vi "Drivetrain Loop.vi"(6 "Reset the clock":bool, 8 "In 4":dbl, 9 "In 3":dbl, 10 "In 2":dbl, 11 "In 1":dbl) -> (0 "Out 4":dbl, 1 "Out 3":dbl, 2 "Out 2":dbl, 3 "Out 1":dbl)   [LabVIEW 2015]
uses:
  Common Code/Drivetrain Modes.ctl
  Robot Global Data.vi
  <vilib>/Rock Robotics/WPI/Solenoid/Deprecated/WPI_SolenoidSetBool.vi
panel:
  out "Modes":T1=enum."Ball Vision Targeting"
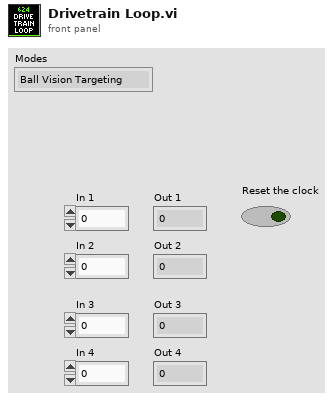
[diagram p1: front panel]
types:
  T1 = typedef "Drivetrain Modes.ctl" = enum16{"Climb", "Manual", "Ball Vision Targeting", "Goal Vision Targeting", "PID Distance Drive", "Hybrid"}
  T2 = typedef "Drivetrain Commands.ctl" = cluster{"Y Power":dbl, "Turn Power":dbl, "1st Gear?":bool, "Modes":T1, "Heading Target":dbl, "X Max Speed":dbl, "Y Max Speed":dbl, "X Min Speed":dbl, "Y Min Speed":dbl, "Y Target":dbl, "Max Accel":dbl, "Max Velocity":dbl}
  T3 = typedef "Dashboard Control Data.ctl" = cluster{"Shooter Presets":T4, "Encoder Control":T6, "Steer PID output":cluster{"output high":dbl, "output low":dbl}, " Steer PID gains":cluster{"proportional gain (Kc)":dbl, "integral time (Ti, min)":dbl, "derivative time (Td, min)":dbl}, "Drivetrain Settings":T7, "Vision Packet":T8, "Dashboard Drivetrain Command":T9, "Info/Command Cluster":T11, "Ball Vision Packet":T12, "Intake Presets":T14, "Intake Encoder Control":T16, "Climb Presets":T17, "Ultrasonic Limit":dbl, "Roll Limit":dbl, "Pitch Limit":dbl, "Goal Output Range":cluster{"output high":dbl, "output low":dbl}}
  T4 = typedef "Shooter Presets.ctl" = cluster{"Batter Shot":T5, "Deep Middle Shot":T5, "Manual Shot":T5, "Left Ticks Per Rotation":dbl, "Right Ticks Per Rotation":dbl, "Low Bar Shot":T5, "Shooter RPM Tolerance":dbl, "IIR Filter Power":dbl, "Trigger Power":dbl, "Fire from Load Delay":i32, "Angle Pot M":dbl, "Angle Pot B":dbl, "Shooter Length":dbl, "String Pot Dist":dbl, "Angle PID gains":cluster{"proportional gain (Kc)":dbl, "integral time (Ti, min)":dbl, "derivative time (Td, min)":dbl}, "Angle Motor Output":cluster{"output high":dbl, "output low":dbl}, "Shooter Angle Tolerance":dbl, "Vision Shoot x^2":dbl, "Vision Shoot x":dbl, "Dist from Axis Cam to Pivot":dbl, "High Goal Center Height":dbl, "Feed Forward Max Accel":dbl, "Feed Forward Kv":dbl, "Backwards Trigger":dbl, "Shot Finish Delay (ms)":dbl, "Angle Max Current":dbl, "Angle Current Trip Time":dbl, "Shooter Intake Angle":dbl, "Vision Shoot c":dbl, "Reset?":bool, "Servo Release Delay":dbl, "Servo Idle Angle":i32, "Servo Hold Angle":i32, "Angle Pot x^2":dbl, "Angle Pot x":dbl, "Angle Pot c":dbl, "Ignore Angle?":bool}
  T5 = typedef "Shot Presets.ctl" = cluster{"Left Wheel RPM":dbl, "Right Wheel RPM":dbl, "Angle":dbl}
  T6 = typedef "Encoder Control.ctl" = cluster{"Right Tick Constant":dbl, "Left Tick Constant":dbl, "Reset?":bool, "Y Dist":cluster{"PID gains":cluster{"proportional gain (Kc)":dbl, "integral time (Ti, min)":dbl, "derivative time (Td, min)":dbl}}, "Y Stop Thresh":dbl, "Y Stop Speed":dbl}
  T7 = typedef "Drivetrain Settings.ctl" = cluster{"Gyro Tolerance":dbl, "Throttle Ramp (ms)":dbl, "Angular rate compensation":bool, "Throttle to Rate Scale":dbl, "Rate compensation gain":dbl, "Kv":dbl, "Ka":dbl, "Feed Forward P":dbl, "Feed Forward D":dbl, "Goal Vision PID gains":cluster{"proportional gain (Kc)":dbl, "integral time (Ti, min)":dbl, "derivative time (Td, min)":dbl}, "Goal Detection Window":dbl}
  T8 = typedef "Goal Vision Packet.ctl" = cluster{"Distance":dbl, "Center X":dbl, "Center Y":dbl, "Found Target?":bool}
  T9 = typedef "Dashboard Drivetrain Command.ctl" = cluster{"Drivetrain Vision":T10}
  T10 = typedef "Drivetrain Vision.ctl" = cluster{"Goal Window":dbl, "Ball Window":dbl}
  T11 = typedef "Ball Tracking Command Cluster.ctl" = cluster{"Distance to Ball":dbl, "Desired Angle":dbl, "Command":enum16{"Turn to Ball", "Turn to Angle", "Get Distance"}, "Pixels from Center":dbl}
  T12 = typedef "Ball Vision Packet.ctl" = cluster{"Ball Detected?":bool, "Distance to Ball":dbl, "Desired Angle":dbl, "Pixels from Center":dbl, "Tracking mode":T13}
  T13 = typedef "Tracking Mode.ctl" = enum16{"Turn to Ball", "Turn to Angle"}
  T14 = typedef "Intake Presets.ctl" = cluster{"Intake Speed":dbl, "Outake Speed":dbl, "Low Height":dbl, "Half Height":dbl, "Full Height":dbl, "Angle Speed":dbl, "Fast Angle":dbl, "Encoder Scale":dbl, "Load Height":dbl, "Output Range":T15, "Rotation Power Max/Min":dbl, "MaxCurrent":dbl, "Intake Trip Time":dbl, "Idle Height":dbl, "Max Height":dbl, "Reset Encoders?":bool, "PID gains":cluster{"proportional gain (Kc)":dbl, "integral time (Ti, min)":dbl, "derivative time (Td, min)":dbl}}
  T15 = typedef "Drivetrain Output Range.ctl" = cluster{"output high":dbl, "output low":dbl}
  T16 = typedef "IntakeEcoderControl.ctl" = cluster{"Arm Tick Constant":dbl, "Reset?":bool, "Y Dist":cluster{"PID gains":cluster{"proportional gain (Kc)":dbl, "integral time (Ti, min)":dbl, "derivative time (Td, min)":dbl}}, "Y Stop Thresh":dbl, "Y Stop Speed":dbl}
  T17 = typedef "Climb Presets.ctl" = cluster{"Pull Power":dbl, "Unpin Power":dbl, "Time to Hold":dbl}
  T18 = typedef "WPI_SolenoidDevRef.ctl" = cluster{"DevStatus":errorcluster, "Pneumatics Control Module":u8, "Forward Solenoid Channel":T19, "Reverse Solenoid Channel":T19}
  T19 = typedef "WPI_SolenoidChannel.ctl" = enum8{"Solenoid 0", "Solenoid 1", "Solenoid 2", "Solenoid 3", "Solenoid 4", "Solenoid 5", "Solenoid 6", "Solenoid 7", "Invalid"}
  T20 = typedef "Dist Drive Status.ctl" = cluster{"Y In Range":bool, "X In Range":bool, "Gyro In Range":bool, "Y Dist":dbl, "X Dist":dbl, "Gyro":dbl}
  T21 = typedef "WPI_MotorControlDeviceRef.ctl" = cluster{"DeviceStatus":errorcluster, "Type":T22, "PWM":cluster{"PWM Channel":T23, "DeadBand":T24}, "CAN":cluster{"Device Number":u8, "Control Mode":T25, "Semaphore":T26, "Max Vout":dbl, "TalonSRX Control Mode":T27}, "Invert":bool}
  T22 = typedef "WPI_MotorControlType.ctl" = enum16{"PWM", "CAN", "CANTalonSRX"}
  T23 = typedef "FPGA_DIOPWMChannel.ctl" = enum8{"PWM 0", "PWM 1", "PWM 2", "PWM 3", "PWM 4", "PWM 5", "PWM 6", "PWM 7", "PWM 8", "PWM 9", "PWM MXP 0", "PWM MXP 1", "PWM MXP 2", "PWM MXP 3", "PWM MXP 4", "PWM MXP 5", "PWM MXP 6", "PWM MXP 7", "PWM MXP 8", "PWM MXP 9", "Invalid"}
  T24 = typedef "WPI_PWMDeadband.ctl" = cluster{"Name":string, "maxPositivePwm":i32, "minPositivePwm":i32, "centerPwm":i32, "maxNegativePwm":i32, "minNegativePwm":i32, "angularRange":u16}
  T25 = typedef "WPI_CANJaguar_ControlMode.ctl" = enum8{"Percent VBus", "Current", "Speed", "Position", "Voltage"}
  T26 = typedef "Semaphore RefNum" = refnum<k1>
  T27 = typedef "WPI_CANTalonSRX_APIControlMode.ctl" = enum8{"Percent VBus", "Speed", "Position", "Slave", "Unchanged / Invalid", "Voltage Compensation", "Current", "Motion Profile"}
  T28 = typedef "Drivetrain Status Cluster.ctl" = cluster{"Modes":T1, "Y (Throttle)":dbl, "X (Steer)":dbl, "Gyro In Range?":bool, "Distance Drive Finished?":bool, "Stop Eject Lockout":bool, "Dist Drive Status":T20, "Y Target":dbl, "Heading Target":dbl, "Vision Target Aligned?":bool, "Gear":dbl, "1st Gear Time":dbl, "2nd Gear Time":dbl, "1st Gear Shifts":dbl, "2nd Gear Shifts":dbl}
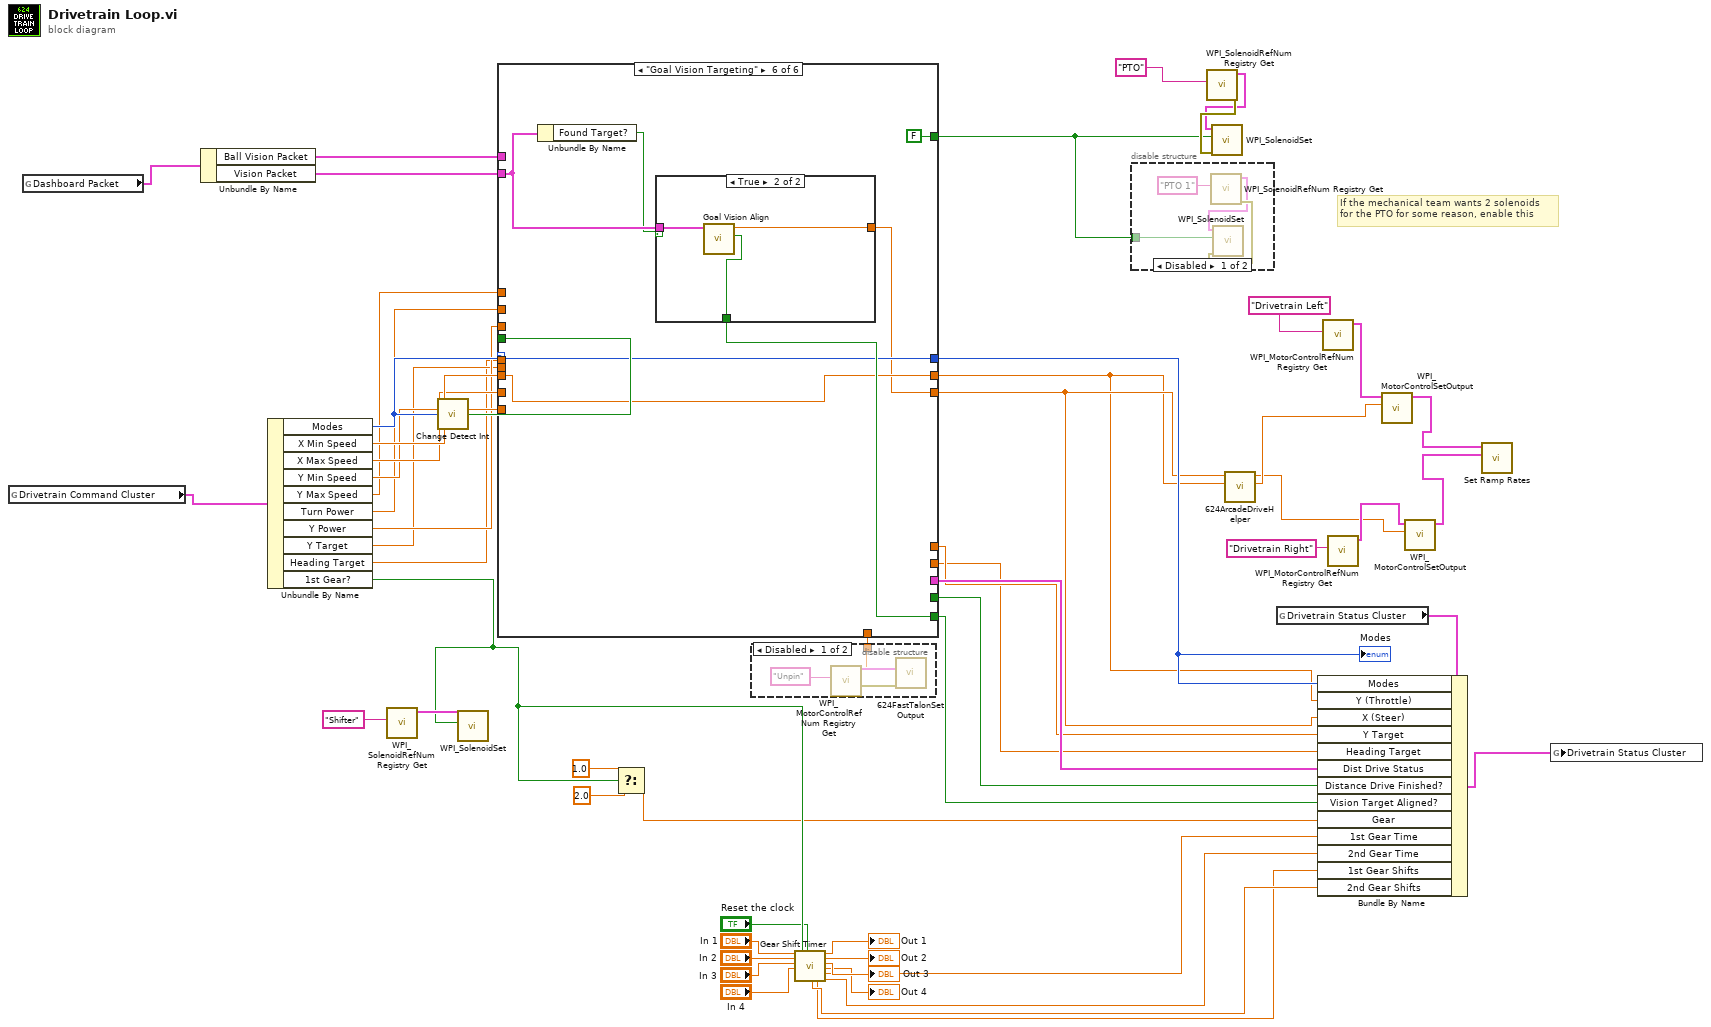
[diagram p0: block diagram]
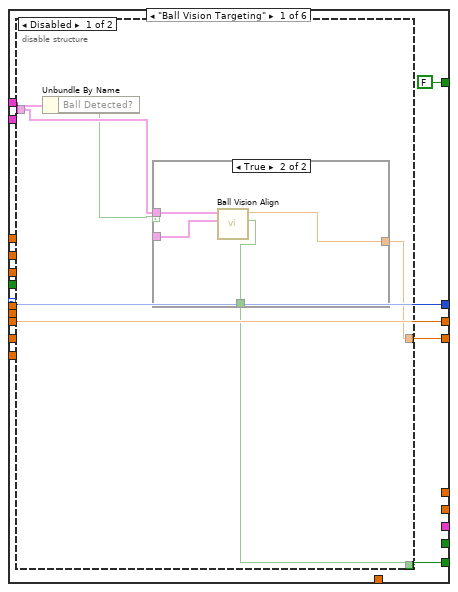
[diagram p3: hidden frame]
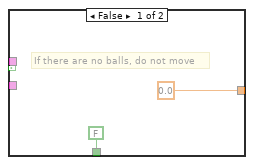
[diagram p4: hidden frame]
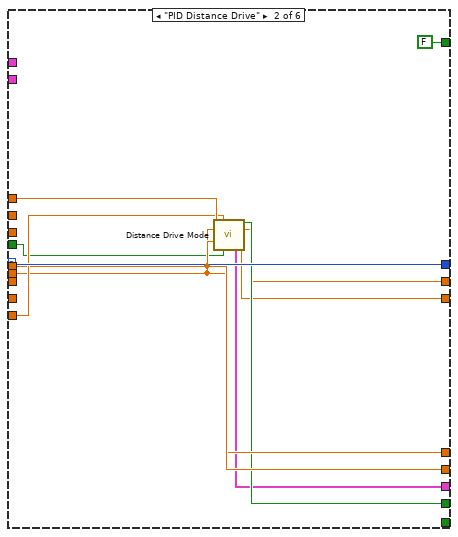
[diagram p6: hidden frame]
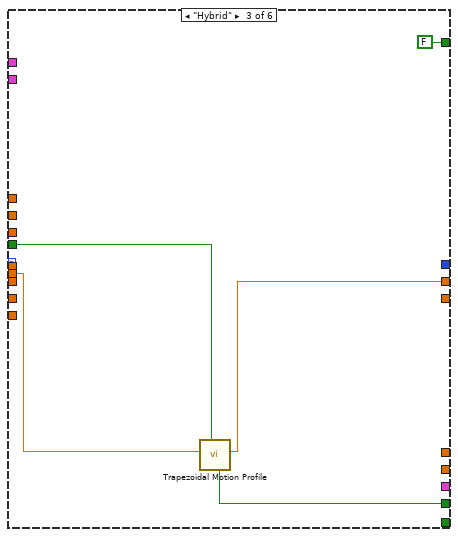
[diagram p7: hidden frame]
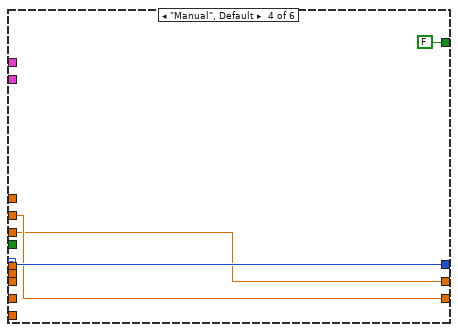
[diagram p8: hidden frame]
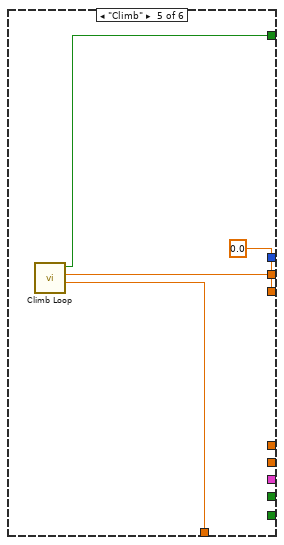
[diagram p9: hidden frame]
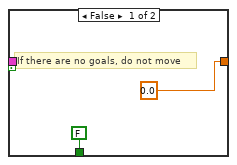
[diagram p10: hidden frame]
diagram:
  # "If the mechanical team wants 2 solenoids\nfor the PTO for some reason, enable this"
  n1 = global read "Robot Global Data.vi" "Drivetrain Command Cluster"() -> (w38:T2)
  n2 = global read "Robot Global Data.vi" "Dashboard Packet"() -> (w11:T3)
  n3 = Unbundle By Name(w11) -> ("Ball Vision Packet"=w13:T12, "Vision Packet"=w12:T8)
  n4 = Unbundle By Name(w38) -> ("Modes"=w48:T1, "X Min Speed"=w47:dbl, "X Max Speed"=w46:dbl, "Y Min Speed"=w45:dbl, "Y Max Speed"=w44:dbl, "Turn Power"=w43:dbl, "Y Power"=w42:dbl, "Y Target"=w41:dbl, "Heading Target"=w40:dbl, "1st Gear?"=w39:bool)
  n5 = call <vilib>:"WPI_SolenoidRefNum Registry Get.vi"("refnum name"="Shifter") -> ("SolenoidDevRef"=w55:T18)  [unwired: 9 in, 1 out]
  n6 = call "Change Detect Int.vi"("In"=w48) -> ("Changed?"=w51:bool)
  n7 = call-poly <vilib>:"WPI_SolenoidSet.vi"("Value"=w39, "SolenoidDevRef"=w55) -> ()  [unwired: 8 in, 2 out]
  n8 = case shown="\"Goal Vision Targeting\"" w48 {
    selector: w48 -> [w61 w84 _ w93 _ w101]
    tunnel: w47 -> [w62 _ _ _ _ w99]
    tunnel: w46 -> [_ _ _ _ _ _]
    tunnel: w45 -> [_ w82 _ _ _ _]
    tunnel: [w62 w77 w89 w91 w95 w99] -> w49
    tunnel: [w59 w75 _ w92 0.0 w98] -> w50
    tunnel: [w61 w84 _ w93 _ w101] -> w54
    tunnel: w51 -> [_ w79 w87 _ _ _]
    tunnel: [w60 _ _ _ _ w102] -> w34
    tunnel: [_ w76 _ _ _ _] -> w32
    tunnel: [_ w78 w88 _ _ _] -> w33
    tunnel: [_ w80 _ _ _ _] -> w31
    tunnel: [_ w81 _ _ _ _] -> w30
    tunnel: w44 -> [_ w83 _ _ _ _]
    tunnel: w43 -> [_ _ _ w92 _ _]
    tunnel: w42 -> [_ _ _ w91 _ _]
    tunnel: w40 -> [_ w81 _ _ _ _]
    tunnel: w41 -> [_ w80 w86 _ _ _]
    tunnel: w13 -> [w58 _ _ _ _ _]
    tunnel: w12 -> [_ _ _ _ _ w104]
    tunnel: [_ _ _ _ w96 _] -> w27
    tunnel: [FALSE ("PTO Engage") FALSE ("PTO Engage") FALSE ("PTO Engage") FALSE ("PTO Engage") w94 FALSE ("PTO Engage")] -> w7
    frame "Ball Vision Targeting" {
      n9 = disable-structure shown="Disabled" {
        disable-tunnel: [w67 _] -> w60
        disable-tunnel: [w66 _] -> w59
        disable-tunnel: w58 -> [w65 _]
        frame Disabled {
          n10 = Unbundle By Name(w65) -> ("Ball Detected?"=w64:bool)
          n11 = case shown="True" w64 {
            tunnel: [0.0 ("Turn Power") w72] -> w66
            tunnel: w65 -> [_ w70]
            tunnel: [FALSE ("Aligned?") w73] -> w67
            tunnel: [_ w71] -> w63
            frame False {
              # "If there are no balls, do not move"
            }
            frame True {
              n12 = call "Ball Vision Align.vi"("Dashboard Drivetrain Command"=w71, "Ball Vision Packet"=w70) -> ("Aligned?"=w73:bool, "Turn Power"=w72:dbl)  [unwired: 8 in]
            }
          }
        }
        frame Enabled {
        }
      }
    }
    frame "PID Distance Drive" {
      n13 = call "Distance Drive Mode.vi"("Y Output High"=w83, "Y Output Low"=w82, "Y target"=w80, "Heading target"=w81, "Reinitialize"=w79) -> ("isFinished"=w78:bool, "Y out"=w77:dbl, "Dist Drive Status"=w76:T20, "X out"=w75:dbl)  [unwired: 7 in]
    }
    frame "Hybrid" {
      n14 = call "Trapezoidal Motion Profile.vi"("Reset?"=w87, "Distance"=w86) -> ("Throttle Out"=w89:sgl, "Finished?"=w88:bool)  [unwired: 8 in]
    }
    frame "Manual", Default {
    }
    frame "Climb" {
      n15 = call "Climb Loop.vi"() -> ("Unpin Power"=w96:dbl, "Pull Power"=w95:dbl, "PTO Engaged?"=w94:bool)  [unwired: 9 in]
    }
    frame "Goal Vision Targeting" {
      n16 = Unbundle By Name(w104) -> ("Found Target?"=w103:bool)
      n17 = case shown="True" w103 {
        tunnel: [0.0 ("Turn Power") w107] -> w98
        tunnel: w104 -> [_ w109]
        tunnel: [FALSE ("Aligned?") w108] -> w102
        frame False {
          # "If there are no goals, do not move"
        }
        frame True {
          n18 = call "Goal Vision Align.vi"("Goal Vision Packet"=w109) -> ("Aligned?"=w108:bool, "Turn Power"=w107:dbl)  [unwired: 9 in]
        }
      }
    }
  }
  "Modes" <- w54
  n19 = Select(t=1.0, s=w39, f=2.0) -> (s? t:f=w29:dbl)
  n20 = disable-structure shown="Disabled" {
    disable-tunnel: w27 -> [w110 _]
    frame Disabled {
      n21 = call <vilib>:"WPI_MotorControlRefNum Registry Get.vi"("refnum name"="Unpin") -> ("error out"=w111:errorcluster, "MotorControlDevRef"=w112:T21)  [unwired: 9 in]
      n22 = call "624FastTalonSetOutput.vi"("error in (no error)"=w111, "Output"=w110, "MotorControlDevRef"=w112) -> ()  [unwired: 7 in, 2 out]
    }
    frame Enabled {
    }
  }
  n23 = call "Gear Shift Timer.vi"("In 1"="In 1", "In 2"="In 2", "In 3"="In 3", "In 4"="In 4", "1st Gear?"=w39, "RESET THE CLOCKS"="Reset the clock") -> ("2nd Gear Shifts"=w23:dbl, "1st Gear Shifts"=w22:dbl, "Out 1"=→"Out 1":dbl, "Out 2"=→"Out 2":dbl, "Out 3"=→"Out 3":dbl, "Out 4"=→"Out 4":dbl, "1st Gear Time"=w17:dbl, "2nd Gear Time"=w16:dbl)  [unwired: 6 in]
  n24 = disable-structure shown="Disabled" {
    disable-tunnel: w7 -> [w114 _]
    frame Disabled {
      n25 = call <vilib>:"WPI_SolenoidRefNum Registry Get.vi"("refnum name"="PTO 1") -> ("error out"=w116:errorcluster, "SolenoidDevRef"=w115:T18)  [unwired: 9 in]
      n26 = call-poly <vilib>:"WPI_SolenoidSet.vi"("error in (no error)"=w116, "Value"=w114, "SolenoidDevRef"=w115) -> ()  [unwired: 7 in, 2 out]
    }
    frame Enabled {
    }
  }
  n27 = call <vilib>:"WPI_SolenoidRefNum Registry Get.vi"("refnum name"="PTO") -> ("error out"=w10:errorcluster, "SolenoidDevRef"=w9:T18)  [unwired: 9 in]
  n28 = call-poly <vilib>:"WPI_SolenoidSet.vi"("error in (no error)"=w10, "Value"=w7, "SolenoidDevRef"=w9) -> ()  [unwired: 7 in, 2 out]
  n29 = call "624ArcadeDriveHelper.vi"("Y Power"=w49, "Turn Power"=w50) -> ("Left"=w5:dbl, "Right"=w1:dbl)  [unwired: 8 in]
  n30 = global read "Robot Global Data.vi" "Drivetrain Status Cluster"() -> (w28:T28)
  n31 = Bundle By Name(cluster=w28, "Modes"=w54, "Y (Throttle)"=w49, "X (Steer)"=w50, "Y Target"=w31, "Heading Target"=w30, "Dist Drive Status"=w32, "Distance Drive Finished?"=w33, "Vision Target Aligned?"=w34, "Gear"=w29, "1st Gear Time"=w17, "2nd Gear Time"=w16, "1st Gear Shifts"=w22, "2nd Gear Shifts"=w23) -> (w35:T28)
  n32 = call <vilib>:"WPI_MotorControlRefNum Registry Get.vi"("refnum name"="Drivetrain Left") -> ("MotorControlDevRef"=w6:T21)  [unwired: 9 in, 1 out]
  n33 = call <vilib>:"WPI_MotorControlRefNum Registry Get.vi"("refnum name"="Drivetrain Right") -> ("MotorControlDevRef"=w3:T21)  [unwired: 9 in, 1 out]
  n34 = call <vilib>:"WPI_MotorControlSetOutput.vi"("Output"=w5, "MotorControlDevRef"=w6) -> ("MotorControlDevRef"=w4:T21)  [unwired: 7 in, 2 out]
  n35 = call <vilib>:"WPI_MotorControlSetOutput.vi"("Output"=w1, "MotorControlDevRef"=w3) -> ("MotorControlDevRef"=w2:T21)  [unwired: 7 in, 2 out]
  n36 = call "Set Ramp Rates.vi"("CAN Talon SRX Ref"=w2, "CAN Talon SRX Ref 2"=w4) -> ()  [unwired: 10 in]
  n37 = global write "Robot Global Data.vi" "Drivetrain Status Cluster"(w35) -> ()
